vi "Twin Shock Filter.vi"() -> ()   [LabVIEW 2015]
uses:
  DIR GAME.ctl
  GAME CLUST.ctl
  <vilib>/Utility/inputDevices.llb/closeKeyboard.vi
  <vilib>/Utility/inputDevices.llb/closeJoystick.vi
panel:
  in  "Target IPAddress":string
  in  "Stop":bool
  in  "Shared Variable??":bool=TRUE
  out "Boolean 2":T1
  out "Start":bool
  in  "Abort":bool
  in  "Claw":bool
  in  "Elbow":bool
  in  "Shoulder":bool
  in  "Base":bool
  out "Direction 2":T2
  out "Claw Motor 2":u32(slide) scale=0.0..100.0
  out "Elbow Motor 2":u32(slide)=50 scale=0.0..100.0
  out "Shoulder Motor 2":u32(slide)=50 scale=0.0..100.0
  out "Base Motor 2":u32(slide)=50 scale=0.0..100.0
  out "Boolean":T3
  out "Direction":T2
  out "Claw Motor":u32(slide) scale=0.0..100.0
  out "Elbow Motor":u32(slide)=50 scale=0.0..100.0
  out "Shoulder Motor":u32(slide)=50 scale=0.0..100.0
  out "Base Motor":u32(slide)=50 scale=0.0..100.0
  # "Arm Controls"
  # "Arm Controls"
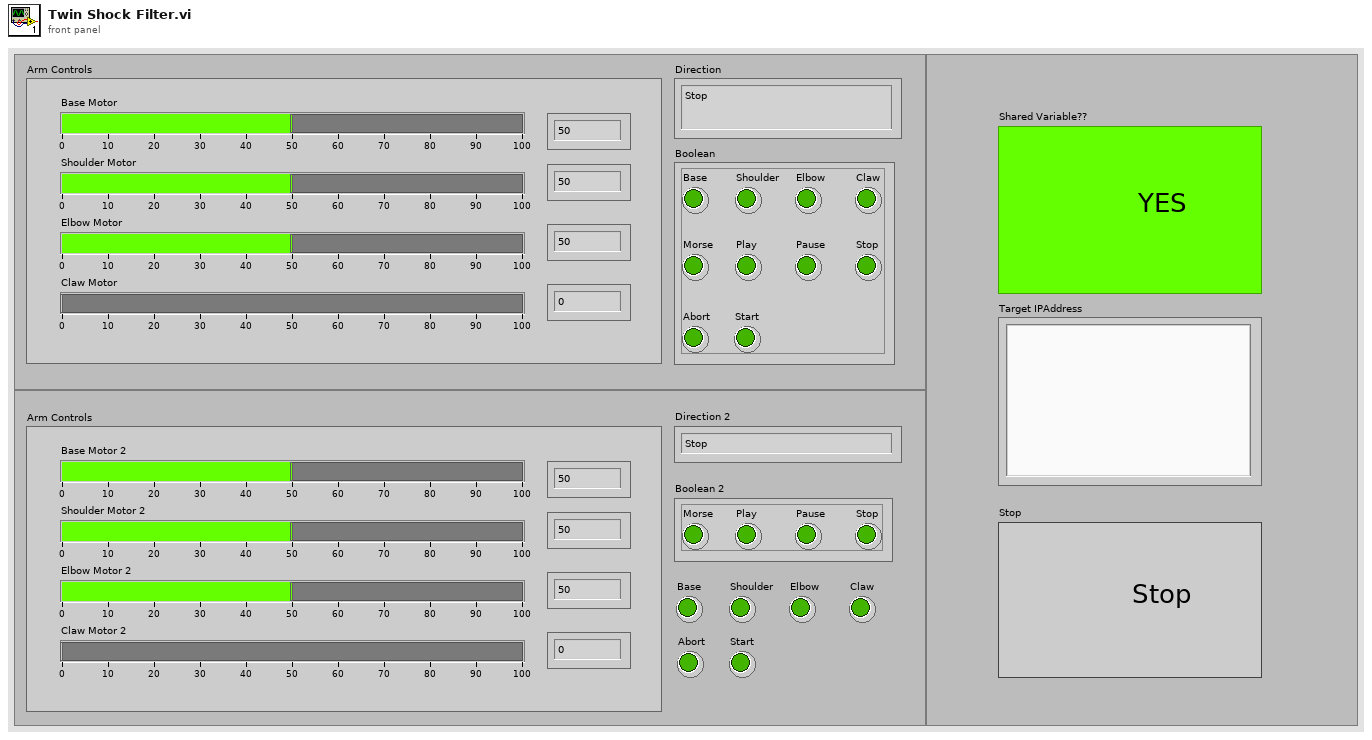
[diagram p1: front panel]
types:
  T1 = cluster{"Morse":bool, "Play":bool, "Pause":bool, "Stop":bool}
  T2 = typedef "DIR GAME.ctl" = enum16{"Stop", "Front", "FR", "Right", "BR", "Back", "BL", "Left", "FL"}
  T3 = typedef "GAME CLUST.ctl" = cluster{"Base":bool, "Shoulder":bool, "Elbow":bool, "Claw":bool, "Morse":bool, "Play":bool, "Pause":bool, "Stop":bool, "Abort":bool, "Start":bool}
  T4 = enum32{"Invalid", "Standard", "Closed", "Hidden", "Minimized", "Maximized"}
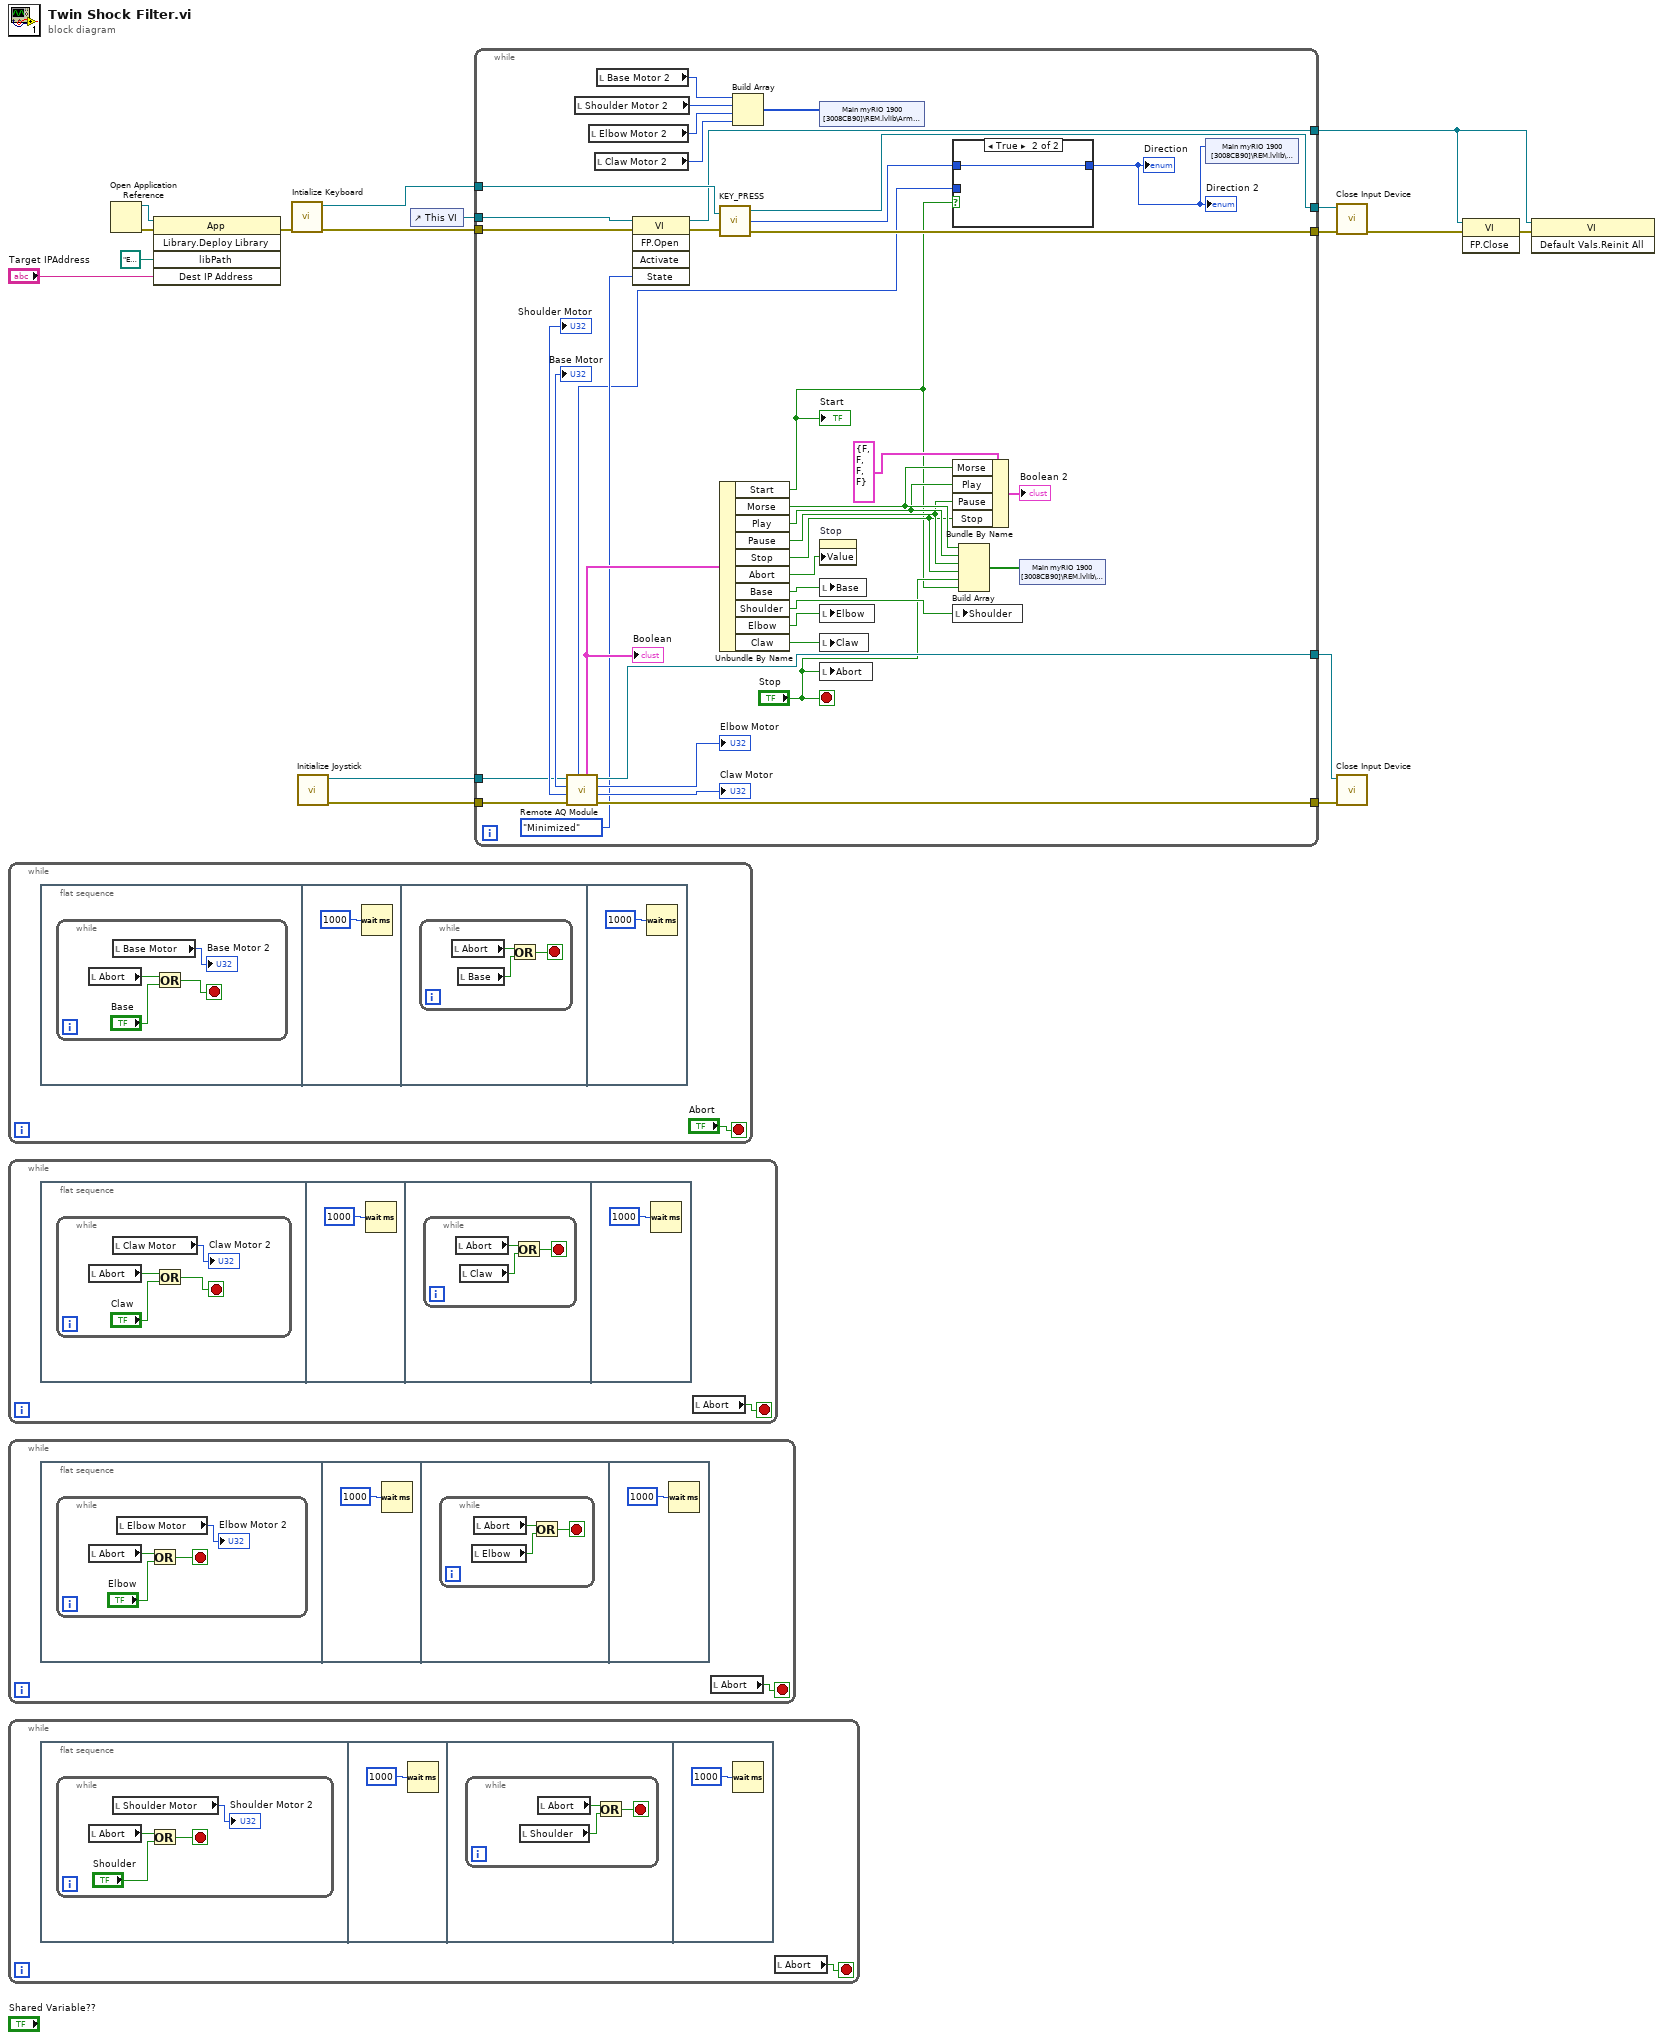
[diagram p0: block diagram]
diagram:
  n1 = while {
    stop <- "Abort" stop-if-true
    n2 = flat-sequence {
      frame #0 {
        n3 = while {
          stop <- w22 stop-if-true
          n4 = local read "Abort"() -> (w21:bool)
          n5 = local read "Base Motor"() -> (→"Base Motor 2":u32)
          n6 = Or(x=w21, y="Base") -> (x .or. y?=w22:bool)
        }
      }
      frame #1 {
        n7 = Wait (ms)(milliseconds to wait=u32 1000) -> ()  [unwired: 1 out]
      }
      frame #2 {
        n8 = while {
          stop <- w24 stop-if-true
          n9 = local read "Abort"() -> (w26:bool)
          n10 = local read "Base"() -> (w25:bool)
          n11 = Or(x=w26, y=w25) -> (x .or. y?=w24:bool)
        }
      }
      frame #3 {
        n12 = Wait (ms)(milliseconds to wait=u32 1000) -> ()  [unwired: 1 out]
      }
    }
  }
  n13 = while {
    stop <- w28 stop-if-true
    n14 = flat-sequence {
      frame #0 {
        n15 = while {
          stop <- w32 stop-if-true
          n16 = local read "Abort"() -> (w31:bool)
          n17 = local read "Claw Motor"() -> (→"Claw Motor 2":u32)
          n18 = Or(x=w31, y="Claw") -> (x .or. y?=w32:bool)
        }
      }
      frame #1 {
        n19 = Wait (ms)(milliseconds to wait=u32 1000) -> ()  [unwired: 1 out]
      }
      frame #2 {
        n20 = while {
          stop <- w34 stop-if-true
          n21 = local read "Abort"() -> (w36:bool)
          n22 = local read "Claw"() -> (w35:bool)
          n23 = Or(x=w36, y=w35) -> (x .or. y?=w34:bool)
        }
      }
      frame #3 {
        n24 = Wait (ms)(milliseconds to wait=u32 1000) -> ()  [unwired: 1 out]
      }
    }
    n25 = local read "Abort"() -> (w28:bool)
  }
  n26 = while {
    stop <- w38 stop-if-true
    n27 = flat-sequence {
      frame #0 {
        n28 = while {
          stop <- w42 stop-if-true
          n29 = local read "Abort"() -> (w41:bool)
          n30 = local read "Elbow Motor"() -> (→"Elbow Motor 2":u32)
          n31 = Or(x=w41, y="Elbow") -> (x .or. y?=w42:bool)
        }
      }
      frame #1 {
        n32 = Wait (ms)(milliseconds to wait=u32 1000) -> ()  [unwired: 1 out]
      }
      frame #2 {
        n33 = while {
          stop <- w44 stop-if-true
          n34 = local read "Elbow"() -> (w45:bool)
          n35 = local read "Abort"() -> (w46:bool)
          n36 = Or(x=w46, y=w45) -> (x .or. y?=w44:bool)
        }
      }
      frame #3 {
        n37 = Wait (ms)(milliseconds to wait=u32 1000) -> ()  [unwired: 1 out]
      }
    }
    n38 = local read "Abort"() -> (w38:bool)
  }
  n39 = while {
    stop <- w48 stop-if-true
    n40 = flat-sequence {
      frame #0 {
        n41 = while {
          stop <- w52 stop-if-true
          n42 = local read "Abort"() -> (w51:bool)
          n43 = local read "Shoulder Motor"() -> (→"Shoulder Motor 2":u32)
          n44 = Or(x=w51, y="Shoulder") -> (x .or. y?=w52:bool)
        }
      }
      frame #1 {
        n45 = Wait (ms)(milliseconds to wait=u32 1000) -> ()  [unwired: 1 out]
      }
      frame #2 {
        n46 = while {
          stop <- w54 stop-if-true
          n47 = local read "Shoulder"() -> (w55:bool)
          n48 = local read "Abort"() -> (w56:bool)
          n49 = Or(x=w56, y=w55) -> (x .or. y?=w54:bool)
        }
      }
      frame #3 {
        n50 = Wait (ms)(milliseconds to wait=u32 1000) -> ()  [unwired: 1 out]
      }
    }
    n51 = local read "Abort"() -> (w48:bool)
  }
  n52 = Open Application Reference() -> (0:w14:errorcluster, 3:w15:refnum<vi>)  [unwired: 4 in]
  n53 = invoke class="App" method="Library.Deploy Library"(reference=w15, error in=w14, "libPath"=path "E:/Anuj/Robotics/Level/LabVIEW/Main VIs/LV15/PDMS/Real Time/REM.lvlib" ("Library Path"), "Dest IP Address"="Target IPAddress") -> (error out=w17:errorcluster)  [unwired: 1 in, 4 out]
  n54 = call <vilib>:"Intialize Keyboard.vi"("error in (no error)"=w17) -> ("error out"=w5:errorcluster, "device ID"=w6:refnum<k1>)  [unwired: 9 in]
  n55 = call <vilib>:"Initialize Joystick.vi"() -> ("error out"=w10:errorcluster, "device ID"=w11:refnum<k1>)  [unwired: 10 in]
  n56 = control-ref of="This VI"() -> (w7:refnum<vi>)
  n57 = while {
    tunnel: w11 -> [w92]
    tunnel: w10 -> [w91]
    tunnel: [w90] -> w9
    tunnel: [w89] -> w8
    tunnel: w7 -> [w70]
    tunnel: w6 -> [w69]
    tunnel: w5 -> [w59]
    tunnel: [w68] -> w4
    tunnel: [w67] -> w3
    tunnel: [w58] -> w1
    stop <- "Stop" stop-if-true
    n58 = call "Remote AQ Module.vi"("error in"=w91, "device ID"=w92) -> ("error out"=w89:errorcluster, "Claw Motor"=→"Claw Motor":u32, "Elbow Motor"=→"Elbow Motor":u32, "device ID 2"=w90:refnum<k1>, "Boolean"=w88:T3, "Direction"=w64:T2, "Shoulder Motor"=→"Shoulder Motor":u32, "Base Motor"=→"Base Motor":u32)
    "Boolean" <- w88
    n59 = local read "Shoulder Motor 2"() -> (w79:u32)
    n60 = local read "Elbow Motor 2"() -> (w78:u32)
    n61 = local read "Claw Motor 2"() -> (w77:u32)
    n62 = local read "Base Motor 2"() -> (w80:u32)
    n63 = invoke class="VI" method="FP.Open"(reference=w70, error in=w59, "State"=T4."Minimized") -> (reference out=w58:refnum<vi>, error out=w60:errorcluster)  [unwired: 2 in, 3 out]
    n64 = call "KEY_PRESS.vi"("device ID"=w69, "error in (no error)"=w60) -> ("device ID 2"=w68:refnum<k1>, "Direction 2"=w65:T2, "error out"=w67:errorcluster)
    n65 = Unbundle By Name(w88) -> ("Start"=w66:bool, "Morse"=w76:bool, "Play"=w75:bool, "Pause"=w74:bool, "Stop"=w73:bool, "Abort"=w81:bool, "Base"=w87:bool, "Shoulder"=w86:bool, "Elbow"=w85:bool, "Claw"=w84:bool)
    "Start" <- w66
    n66 = Build Array(w80, w79, w78, w77) -> (w63:u32[])
    n67 = shared-variable "Main myRIO 1900 [3008CB90]\\REM.lvlib\\Arm Values"(w63) -> ()  [unwired: 1 in, 1 out]
    n68 = property on="Stop" class="Bool (strict)"("Value"=w81) -> ()  [unwired: 2 in, 2 out]
    n69 = local write "Base"(w87) -> ()
    n70 = local write "Elbow"(w85) -> ()
    n71 = local write "Claw"(w84) -> ()
    n72 = local write "Abort"("Stop") -> ()
    n73 = case shown="True" w66 {
      tunnel: [w97 w98] -> w61
      tunnel: w65 -> [_ w98]
      tunnel: w64 -> [w97 _]
      frame False {
      }
      frame True {
      }
    }
    "Direction" <- w61
    "Direction 2" <- w61
    n74 = Bundle By Name(cluster=T1 {"Morse"=FALSE, "Play"=FALSE, "Pause"=FALSE, "Stop"=FALSE} ("Boolean 3"), "Morse"=w76, "Play"=w75, "Pause"=w74, "Stop"=w73) -> (→"Boolean 2":T1)
    n75 = local write "Shoulder"(w86) -> ()
    n76 = Build Array(w76, w75, w74, w73, "Stop", w66) -> (w62:bool[])
    n77 = shared-variable "Main myRIO 1900 [3008CB90]\\REM.lvlib\\Buttons"(w62) -> ()  [unwired: 1 in, 1 out]
    n78 = shared-variable "Main myRIO 1900 [3008CB90]\\REM.lvlib\\Direction"(w61) -> ()  [unwired: 1 in, 1 out]
  }
  n79 = call-poly <vilib>:"Close Input Device.vi"("error in (no error)"=w3, "device ID"=w4) -> ("error out"=w16:errorcluster)  [unwired: 8 in]
  n80 = call-poly <vilib>:"Close Input Device.vi"("error in (no error)"=w8, "device ID"=w9) -> ()  [unwired: 8 in, 1 out]
  n81 = invoke class="VI" method="FP.Close"(reference=w1, error in=w16) -> (error out=w2:errorcluster)  [unwired: 1 in, 2 out]
  n82 = invoke class="VI" method="Default Vals.Reinit All"(reference=w1, error in=w2) -> ()  [unwired: 1 in, 3 out]
